vi "qweer.vi"() -> ()   [LabVIEW 2015]
uses:
  Data.ctl
  State.ctl
  <vilib>/rvi/Emulation/niFpgaGetClockAttributes.vi
  <vilib>/rvi/Emulation/niFpgaSctlEmulationGetInTimedLoop.vi
  <vilib>/rvi/Emulation/niFpgaEmulationReportErrorSimple.vi
  <vilib>/rvi/Emulation/niFpgaProcessEmulError.vi
  <vilib>/rvi/Emulation/niFpgaCriticalErrorInLSC.vi
  <vilib>/rvi/eio/common/nirviEmuTemplateMethod_errors.vi
  <vilib>/eio/EIONode/EIONode.xnode
panel:
  out "Data array":i32[](array[numeric])
  in  "stop":bool
  in  "Gain/ChannelSelect":T1(ring)
  in  "PowerDown?":bool
  out "Data":i32
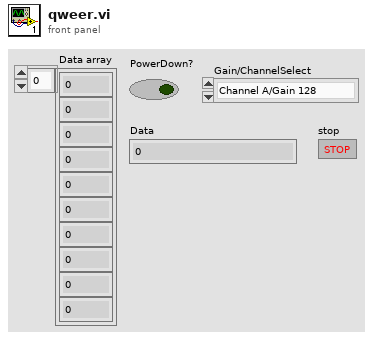
[diagram p1: front panel]
types:
  T1 = enum16{"Channel A/Gain 128", "Channel A/Gain 64", "Channel B/Gain 32"}
  T2 = typedef "State.ctl" = enum16{"PowerUp", "PowerDown", "Gain/ChannelSelect", "ReadData", "ClockLow", "ClockHigh", "ConvertData", "RetrievalReady?"}
  T3 = typedef "Data.ctl" = cluster{"DT":bool, "SCK":bool, "2's Data":i32, "PulseCount":u8, "DelayTime":u8, "Data":i32, "PowerDown?":bool, "Gain/ChannelSelect":enum16{"Channel A/Gain 128", "Channel A/Gain 64", "Channel B/Gain 32"}}
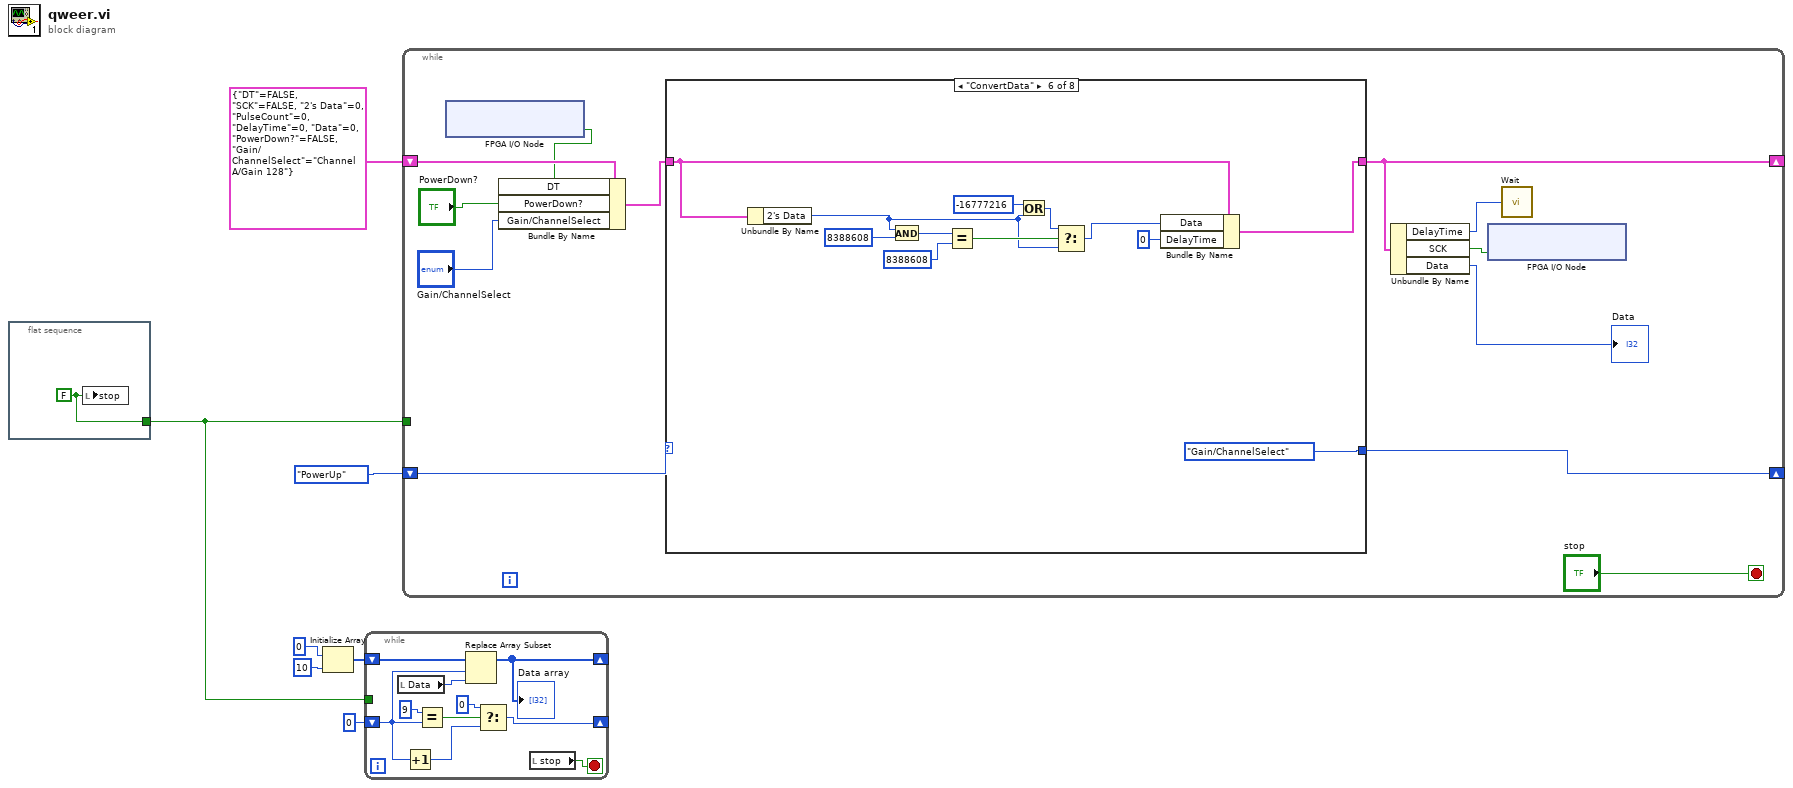
[diagram p0: block diagram]
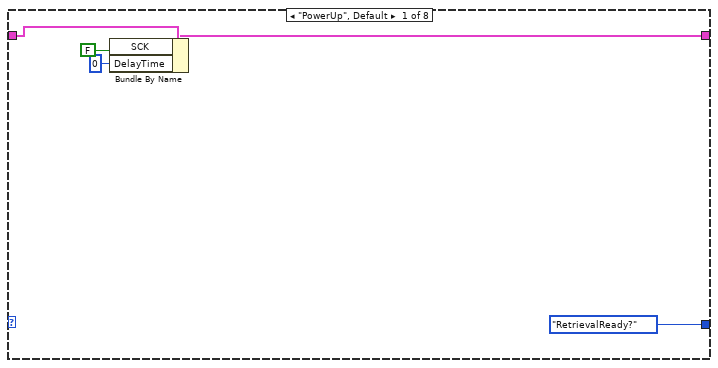
[diagram p2: hidden frame]
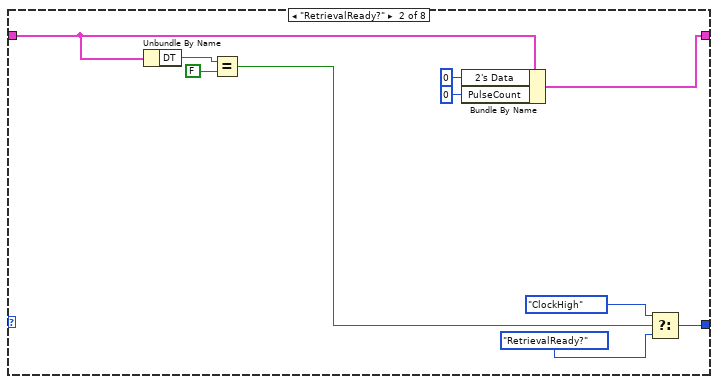
[diagram p3: hidden frame]
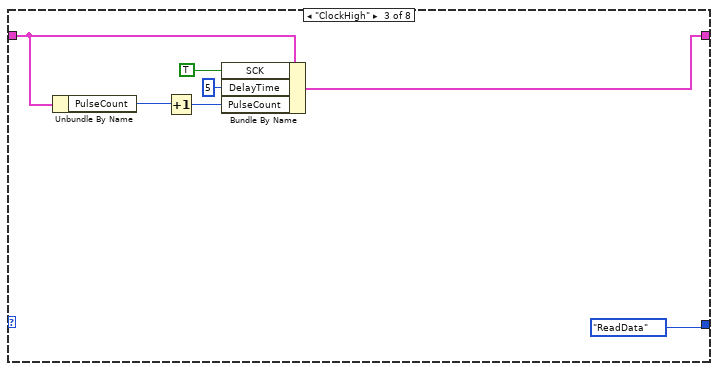
[diagram p4: hidden frame]
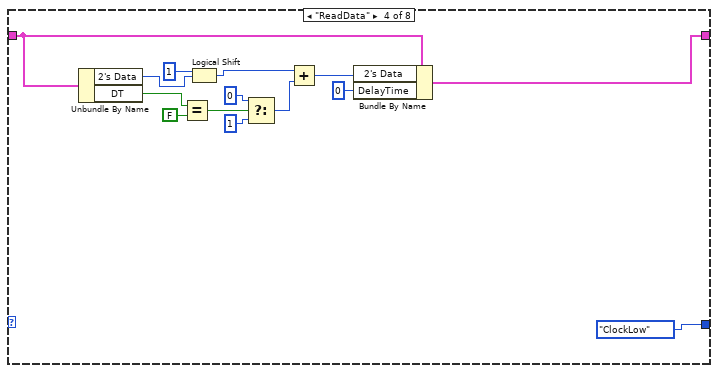
[diagram p5: hidden frame]
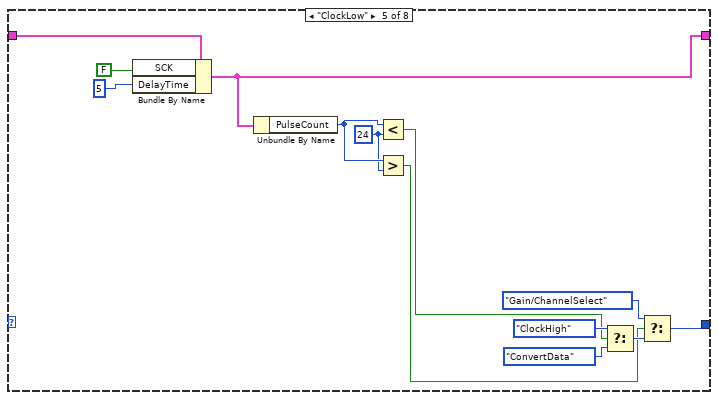
[diagram p6: hidden frame]
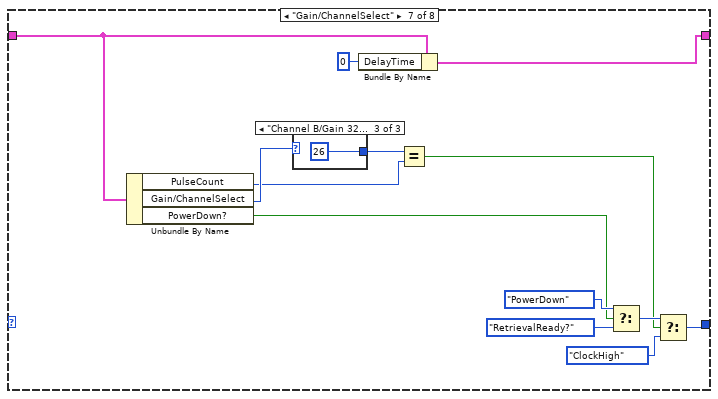
[diagram p7: hidden frame]
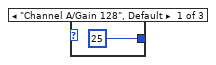
[diagram p8: hidden frame]
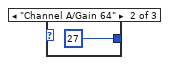
[diagram p9: hidden frame]
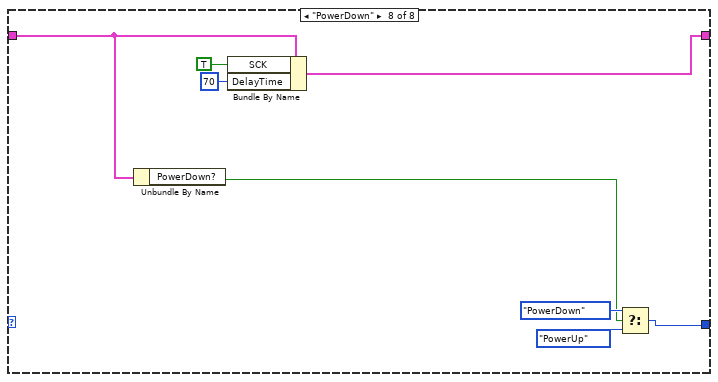
[diagram p10: hidden frame]
diagram:
  n1 = flat-sequence {
    tunnel: [w8] -> w1
    frame #0 {
      w8 = FALSE
      n2 = local write "stop"(w8) -> ()
    }
  }
  n3 = Initialize Array(0 ("Data"), 10 ("dimension size")) -> (w4:i32[])
  n4 = while {
    shift-right: [w10] -> _
    shift-left: w4 -> [w11]
    shift-right: [w16] -> _
    shift-left: 0 ("index") -> [w12]
    tunnel: w1 -> [_]
    stop <- w9 stop-if-true
    n5 = local read "Data"() -> (w18:i32)
    n6 = Increment(x=w12) -> (x+1=w15:i32)
    n7 = Equal?(x=9, y=w12) -> (x = y?=w13:bool)
    n8 = Replace Array Subset(array=w11, new element=w18, index=w12) -> (w10:i32[])
    "Data array" <- w10
    n9 = Select(t=0 ("index"), s=w13, f=w15) -> (s? t:f=w16:i32)
    n10 = local read "stop"() -> (w9:bool)
  }
  n11 = while {
    shift-right: [w21] -> _
    shift-left: T3 {"DT"=FALSE, "SCK"=FALSE, "2's Data"=0, "PulseCount"=0, "DelayTime"=0, "Data"=0, "PowerDown?"=FALSE, "Gain/ChannelSelect"=enum."Channel A/Gain 128"} ("Data") -> [w27]
    shift-right: [w28] -> _
    shift-left: State."PowerUp" ("State") -> [w30]
    tunnel: w1 -> [_]
    stop <- "stop" stop-if-true
    n12 = xnode "FPGA I/O Node"() -> ("ConnectorA/DIO0"=w25:bool)  [unwired: 1 in, 1 out]
    n13 = Bundle By Name(cluster=w27, "DT"=w25, "PowerDown?"="PowerDown?", "Gain/ChannelSelect"="Gain/ChannelSelect") -> (w26:T3)
    n14 = case shown="\"ConvertData\"" w30 {
      tunnel: w26 -> [w35 w39 w48 w53 w79 w84 w94 w109]
      tunnel: [w33 w38 w52 w55 w74 w83 w93 w115] -> w21
      tunnel: [State."RetrievalReady?" ("State") w41 State."ReadData" ("State") State."ClockLow" ("State") w75 State."Gain/ChannelSelect" ("State") w101 w110] -> w28
      frame "PowerUp", Default {
        n15 = Bundle By Name(cluster=w35, "SCK"=FALSE, "DelayTime"=u8 0) -> (w33:T3)
      }
      frame "RetrievalReady?" {
        n16 = Unbundle By Name(w39) -> ("DT"=w45:bool)
        n17 = Equal?(x=w45, y=FALSE) -> (x = y?=w40:bool)
        n18 = Bundle By Name(cluster=w39, "2's Data"=0, "PulseCount"=u8 0) -> (w38:T3)
        n19 = Select(t=State."ClockHigh" ("State"), s=w40, f=State."RetrievalReady?" ("State")) -> (s? t:f=w41:T2)
      }
      frame "ClockHigh" {
        n20 = Unbundle By Name(w48) -> ("PulseCount"=w47:u8)
        n21 = Increment(x=w47) -> (x+1=w46:u8)
        n22 = Bundle By Name(cluster=w48, "SCK"=TRUE, "DelayTime"=u8 5, "PulseCount"=w46) -> (w52:T3)
      }
      frame "ReadData" {
        n23 = Unbundle By Name(w53) -> ("2's Data"=w66:i32, "DT"=w64:bool)
        n24 = Equal?(x=w64, y=FALSE ("SCK")) -> (x = y?=w62:bool)
        n25 = Logical Shift(y=i16 1, x=w66) -> (x << y=w61:i32)
        n26 = Select(t=0 ("DelayTime"), s=w62, f=1 ("DelayTime")) -> (s? t:f=w58:i32)
        n27 = Add(x=w61, y=w58) -> (x+y=w57:i32)
        n28 = Bundle By Name(cluster=w53, "2's Data"=w57, "DelayTime"=u8 0) -> (w55:T3)
      }
      frame "ClockLow" {
        w68 = u8 24 ("y")
        n29 = Bundle By Name(cluster=w79, "SCK"=FALSE, "DelayTime"=u8 5) -> (w74:T3)
        n30 = Unbundle By Name(w74) -> ("PulseCount"=w69:u8)
        n31 = Less?(x=w69, y=w68) -> (x < y?=w71:bool)
        n32 = Greater?(x=w69, y=w68) -> (0:w67:bool)
        n33 = Select(t=State."ClockHigh" ("State"), s=w71, f=State."ConvertData" ("State")) -> (s? t:f=w70:T2)
        n34 = Select(t=State."Gain/ChannelSelect" ("State"), s=w67, f=w70) -> (s? t:f=w75:T2)
      }
      frame "ConvertData" {
        n35 = Unbundle By Name(w84) -> ("2's Data"=w85:i32)
        n36 = And(x=w85, y=8388608) -> (x .and. y?=w90:i32)
        n37 = Equal?(x=w90, y=8388608) -> (x = y?=w88:bool)
        n38 = Or(x=-16777216 ("y"), y=w85) -> (x .or. y?=w86:i32)
        n39 = Select(t=w86, s=w88, f=w85) -> (s? t:f=w81:i32)
        n40 = Bundle By Name(cluster=w84, "Data"=w81, "DelayTime"=u8 0) -> (w83:T3)
      }
      frame "Gain/ChannelSelect" {
        n41 = Unbundle By Name(w94) -> ("PulseCount"=w97:u8, "Gain/ChannelSelect"=w99:T1, "PowerDown?"=w100:bool)
        n42 = case shown="\"Channel B/Gain 32\"" w99 {
          tunnel: [u8 25 ("PulseCount") u8 27 ("PulseCount") u8 26 ("PulseCount")] -> w98
          frame "Channel A/Gain 128", Default {
          }
          frame "Channel A/Gain 64" {
          }
          frame "Channel B/Gain 32" {
          }
        }
        n43 = Bundle By Name(cluster=w94, "DelayTime"=u8 0) -> (w93:T3)
        n44 = Equal?(x=w98, y=w97) -> (x = y?=w95:bool)
        n45 = Select(t=State."PowerDown" ("State"), s=w100, f=State."RetrievalReady?" ("State")) -> (s? t:f=w96:T2)
        n46 = Select(t=w96, s=w95, f=State."ClockHigh" ("State")) -> (s? t:f=w101:T2)
      }
      frame "PowerDown" {
        n47 = Unbundle By Name(w109) -> ("PowerDown?"=w108:bool)
        n48 = Bundle By Name(cluster=w109, "SCK"=TRUE, "DelayTime"=u8 70) -> (w115:T3)
        n49 = Select(t=State."PowerDown" ("State"), s=w108, f=State."PowerUp" ("State")) -> (s? t:f=w110:T2)
      }
    }
    n50 = Unbundle By Name(w21) -> ("DelayTime"=w29:u8, "SCK"=w20:bool, "Data"=→"Data":i32)
    n51 = xnode "FPGA I/O Node"("ConnectorA/DIO8"=w20) -> ()  [unwired: 1 in, 1 out]
    n52 = call "Wait"("Count(uSec)"=w29) -> ()  [unwired: 1 out]
  }
